vi "normalize_array_advanced_float.vi"(10 "i32_ar_first_and_last_pixel":i32[](array[numeric]), 11 "unwrapped array":dbl[](array[numeric])) -> (0 "norm factor":dbl, 1 "offset":i16, 2 "i16_normalized unwrapped array":dbl[](array[numeric]), 3 "normalized unwrapped array":u8[](array[numeric]), 4 "normalizing part":i16[](array[numeric]))   [LabVIEW 2011]
doc: "Normalizes the row to values between 0 and 255 as well as set the mask values to zero."
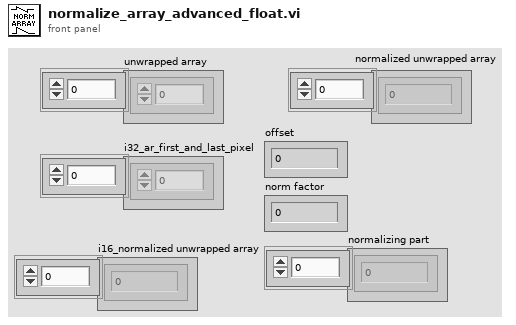
[diagram p1: front panel]
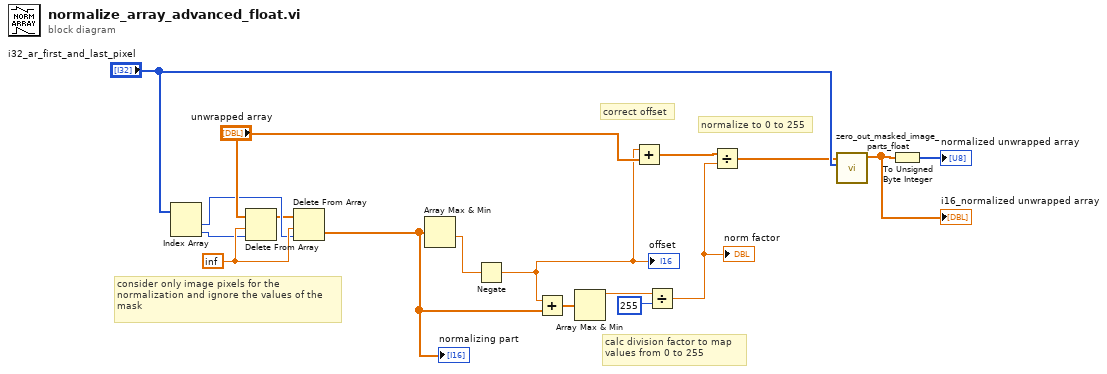
[diagram p0: block diagram]
diagram:
  w9 = inf
  # "normalize to 0 to 255"
  # "calc division factor to map\nvalues from 0 to 255"
  # "consider only image pixels for the \nnormalization and ignore the values of the\nmask"
  # "correct offset"
  n1 = Index Array(array="i32_ar_first_and_last_pixel") -> (element #1=w8:i32, element #2=w3:i32)  [unwired: 2 in]
  n2 = Delete From Array(array="unwrapped array", length=w9, index=w3) -> (array with subset deleted=w7:dbl[])  [unwired: 1 out]
  n3 = Delete From Array(array=w7, length=w9, index=w8) -> (deleted portion=w11:dbl[])  [unwired: 1 out]
  "normalizing part" <- w11
  n4 = Array Max & Min(array=w11) -> (min value=w10:dbl)  [unwired: 3 out]
  n5 = Negate(x=w10) -> (-x=w4:dbl)
  "offset" <- w4
  n6 = Add(x=w4, y=w11) -> (x+y=w14:dbl[])
  n7 = Array Max & Min(array=w14) -> (max value=w13:dbl)  [unwired: 3 out]
  n8 = Add(x=w4, y="unwrapped array") -> (x+y=w16:dbl[])
  n9 = Divide(x=w13, y=i16 255) -> (x/y=w17:dbl)
  "norm factor" <- w17
  n10 = Divide(x=w16, y=w17) -> (x/y=w2:dbl[])
  n11 = call "zero_out_masked_image_parts_float.vi"("i32_ar_first_and_last_pixel"="i32_ar_first_and_last_pixel", "unwrapped_Array"=w2) -> ("Array out"=w1:dbl[])  [unwired: 9 in]
  "i16_normalized unwrapped array" <- w1
  n12 = To Unsigned Byte Integer(number=w1) -> (unsigned 8bit integer=→"normalized unwrapped array":u8[])
